vi "Stop Live Mode.vi"(8 "error in (no error)":errorcluster, 11 "Orca-Flash 4.0 V2 in":refnum<class "Hamamatsu Camera.lvclass">) -> (0 "error out":errorcluster, 3 "Orca-Flash 4.0 V2 out":refnum<class "Hamamatsu Camera.lvclass">)   [LabVIEW 2022 SP3, in "Hamamatsu Camera.lvlib" / "Hamamatsu Camera.lvclass"]
uses:
  Hamamatsu Camera.lvclass
  Hamamatsu Camera.lvclass/Hamamatsu Camera.ctl
  Camera/Camera.lvclass
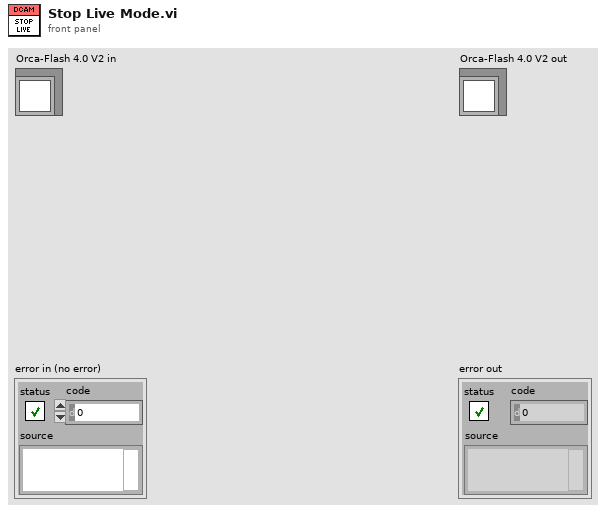
[diagram p1: front panel]
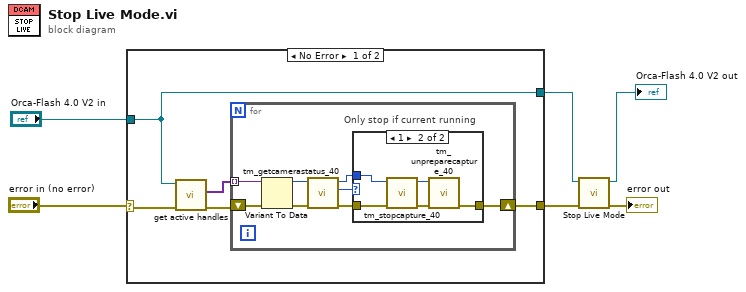
[diagram p0: block diagram]
diagram:
  n1 = case shown="No Error" "error in (no error)" {
    selector: "error in (no error)" -> [w9 w27]
    tunnel: "Orca-Flash 4.0 V2 in" -> [w8 w26]
    tunnel: [w8 w26] -> w2
    tunnel: [w11 w27] -> w3
    frame No Error {
      n2 = call-dynamic "get active handles.vi"("error in (no error)"=w9, "Camera in"=w8) -> ("error out"=w10:errorcluster, "Handles"=w7:variant[])  [unwired: 5 in, 3 out]
      n3 = for {
        tunnel: w7 -> [w13] mode=indexing
        shift-right: [w19] -> w11
        shift-left: w10 -> [w16]
        # "Only stop if current running"
        n4 = Variant To Data(error in=w16, Variant=w13) -> (data=w14:u32, error out=w15:errorcluster)  [unwired: 1 in]
        n5 = call <userlib>:"tm_getcamerastatus_40.vi"("error in (no error)"=w15, "Handle in"=w14) -> ("error out"=w18:errorcluster, "Status"=w17:i32, "Handle out"=w12:u32)  [unwired: 7 in]
        n6 = case shown="1" w17 {
          tunnel: w12 -> [_ w23]
          tunnel: [w20 w22] -> w19
          tunnel: w18 -> [w20 w21]
          frame Default {
          }
          frame 1 {
            n7 = call <userlib>:"tm_stopcapture_40.vi"("error in (no error)"=w21, "Handle in"=w23) -> ("error out"=w25:errorcluster, "Handle out"=w24:u32)  [unwired: 8 in]
            n8 = call <userlib>:"tm_unpreparecapture_40.vi"("error in (no error)"=w25, "Handle in"=w24) -> ("error out"=w22:errorcluster)  [unwired: 8 in, 1 out]
          }
        }
      }
    }
    frame Error {
    }
  }
  n9 = call-parent "Stop Live Mode.vi"("error in (no error)"=w3, "Camera in"=w2) -> ("error out"=→"error out":errorcluster, "Camera out"=→"Orca-Flash 4.0 V2 out":refnum<class "Hamamatsu Camera.lvclass">)  [unwired: 8 in]
